vi "Combined_Code_V1.vi"() -> ()   [LabVIEW 2015]
panel:
  out "Boolean 2":bool
  out "RPS Value":dbl
  in  "Encoder Rising Simulate":bool
  out "Counts":dbl
  out "millisecond timer value":u32
  out "time elapsed in Frame 1":u32
  in  "Encoder Turn Pulse":bool
  in  "Encoder PPT":dbl
  out "Gauge":dbl(knob) scale=0.0..360.0
  out "Waveform Chart":dbl(graph)
  out "Crank Angle":dbl
  in  "stop 2":bool
  in  "stop":bool
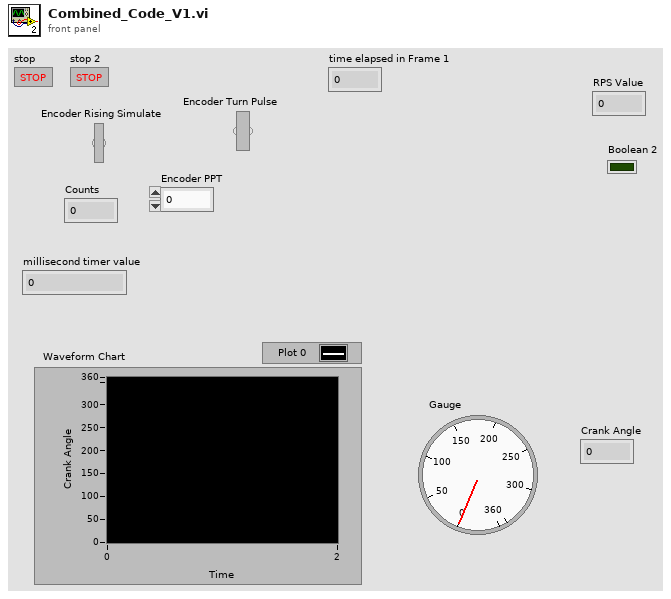
[diagram p1: front panel]
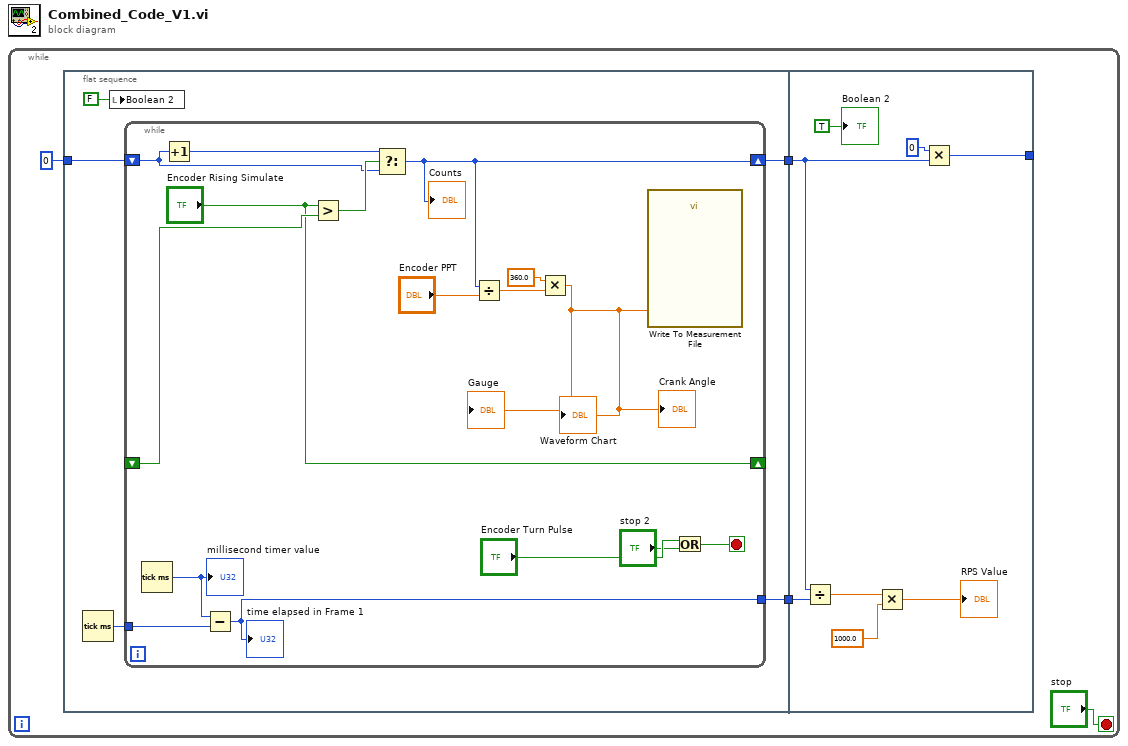
[diagram p0: block diagram]
diagram:
  n1 = while {
    stop <- "stop" stop-if-true
    n2 = flat-sequence {
      tunnel: [w9] -> w4
      tunnel: u8 0 -> [w7]
      tunnel: [w5] -> w2
      tunnel: w4 -> [w26]
      tunnel: w2 -> [w29]
      tunnel: [w28] -> _
      frame #0 {
        n3 = Tick Count (ms)() -> (millisecond timer value=w6:u32)
        n4 = local write "Boolean 2"(FALSE ("Boolean 2")) -> ()
        n5 = while {
          shift-right: ["Encoder Rising Simulate"] -> _
          shift-left: _ -> [w25]
          shift-right: [w11] -> w9
          shift-left: w7 -> [w21]
          tunnel: w6 -> [w19]
          tunnel: [w13] -> w5
          stop <- w12 stop-if-true
          n6 = Tick Count (ms)() -> (millisecond timer value=w20:u32)
          "millisecond timer value" <- w20
          n7 = Increment(x=w21) -> (x+1=w22:u8)
          n8 = Subtract(x=w20, y=w19) -> (x-y=w13:u32)
          "time elapsed in Frame 1" <- w13
          n9 = Greater?(x="Encoder Rising Simulate", y=w25) -> (0:w23:bool)
          n10 = Select(t=w22, s=w23, f=w21) -> (s? t:f=w11:u8)
          "Counts" <- w11
          n11 = Divide(x=w11, y="Encoder PPT") -> (x/y=w17:dbl)
          n12 = Multiply(x=360.0, y=w17) -> (x*y=w10:dbl)
          "Gauge" <- w10
          "Waveform Chart" <- w10
          "Crank Angle" <- w10
          n13 = call "Write To Measurement File"("Signals"=w10) -> ()  [unwired: 16 in, 3 out]
          n14 = Or(x="Encoder Turn Pulse", y="stop 2") -> (x .or. y?=w12:bool)
        }
      }
      frame #1 {
        n15 = Divide(x=w26, y=w29) -> (x/y=w31:dbl)
        n16 = Multiply(x=w31, y=1000.0) -> (x*y=→"RPS Value":dbl)
        n17 = Multiply(x=u8 0, y=w26) -> (x*y=w28:u8)
        "Boolean 2" <- TRUE ("Boolean 2")
      }
    }
  }
